vi "Do.vi"(8 "error in (no error)":errorcluster, 10 "Actor In":refnum<class "Actor.lvclass">, 11 "Last Ack Msg in":refnum<class "Last Ack Msg.lvclass">) -> (0 "error out":errorcluster, 1 "Stop Actor":bool, 2 "Actor Out":refnum<class "Actor.lvclass">)   [LabVIEW 2022 SP3, in "Artifex.lvlib" / "Last Ack Msg.lvclass"]
uses:
  Last Ack Msg.lvclass
  Actor/Actor.lvclass
  Last Ack Msg.lvclass/Last Ack Msg.ctl
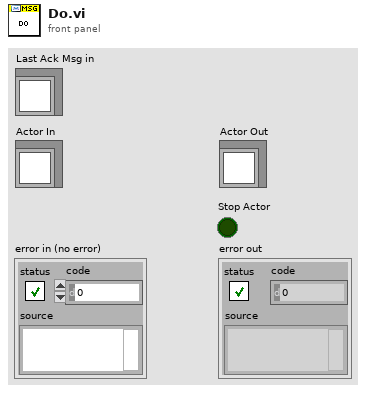
[diagram p1: front panel]
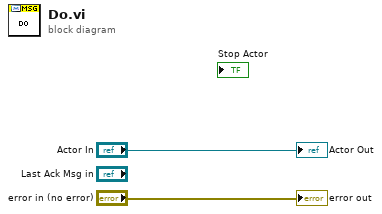
[diagram p0: block diagram]
diagram:
  "error out" <- "error in (no error)"
  "Actor Out" <- "Actor In"
